vi "3D Cartesian Coordinate Shift (Array).vi"(8 "shift":cluster{"dx":dbl, "dy":dbl, "dz":dbl}, 9 "Z":dbl[](array[numeric]), 10 "Y":dbl[](array[numeric]), 11 "X":dbl[](array[numeric])) -> (0 "error":i32, 1 "Z Out":dbl[](array[numeric]), 2 "Y Out":dbl[](array[numeric]), 3 "X Out":dbl[](array[numeric]))   [LabVIEW 2020, in "NI_AALPro.lvlib"]
doc: "Shifts three-dimensional Cartesian coordinates along the x-, y-, and z-axes. \n\nWire data to the <B>X</B> input to determine the polymorphic instance to use or manually select the instance."
uses:
  NI_AALPro.lvlib
  <resource>/lvanlys.dll
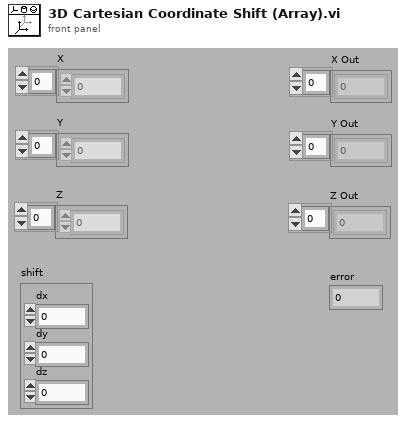
[diagram p1: front panel]
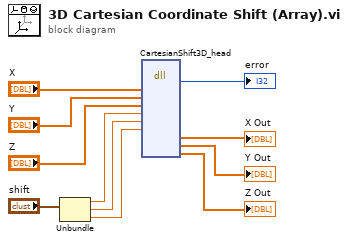
[diagram p0: block diagram]
diagram:
  n1 = Unbundle("shift") -> ("dx"=w7:dbl, "dy"=w6:dbl, "dz"=w5:dbl)
  n2 = dll-call lib="C:/Program Files (x86)/National Instruments/LabVIEW 2020/resource/lvanlys.*" fn="CartesianShift3D_head"("X"="X", "Y"="Y", "Z"="Z", "dx"=w7, "dy"=w6, "dz"=w5) -> (→"error":i32, "Xout"=→"X Out":dbl[], "Yout"=→"Y Out":dbl[], "Zout"=→"Z Out":dbl[])  [unwired: 12 in, 2 out]
